vi "Get all positions.vi"(7 "JSON":string, 9 "Offset":i32) -> (1 "Offset past All":i32, 2 "Array":T2(array[cluster]), 3 "State":T3)   [LabVIEW 2017, in "JSONtext.lvlib"]
uses:
  JSONtext.lvlib
  Parsing State.ctl
  JSON Value Type.ctl
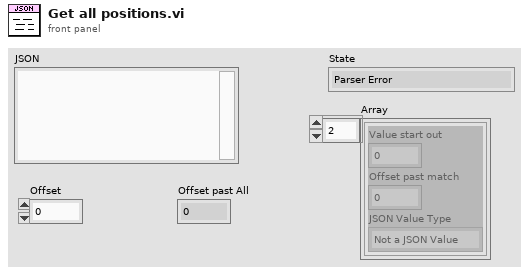
[diagram p1: front panel]
types:
  T1 = typedef "JSONtext.lvlib/JSON Value Type.ctl" = enum16{"Not a JSON Value", "JSON Object", "JSON Array", "String", "Number", "true", "false", "null"}
  T2 = cluster{"Value start out":i32, "Offset past match":i32, "JSON Value Type":T1}[]
  T3 = typedef "JSONtext.lvlib/Parsing State.ctl" = enum16{"Parser Error", "Object", "Array", "String", "Number/Other", "Leading Whitespace", "Object end", "Array end", "Value end"}
  T4 = cluster{"Value start out":i32, "Offset past match":i32, "JSON Value Type":T1}
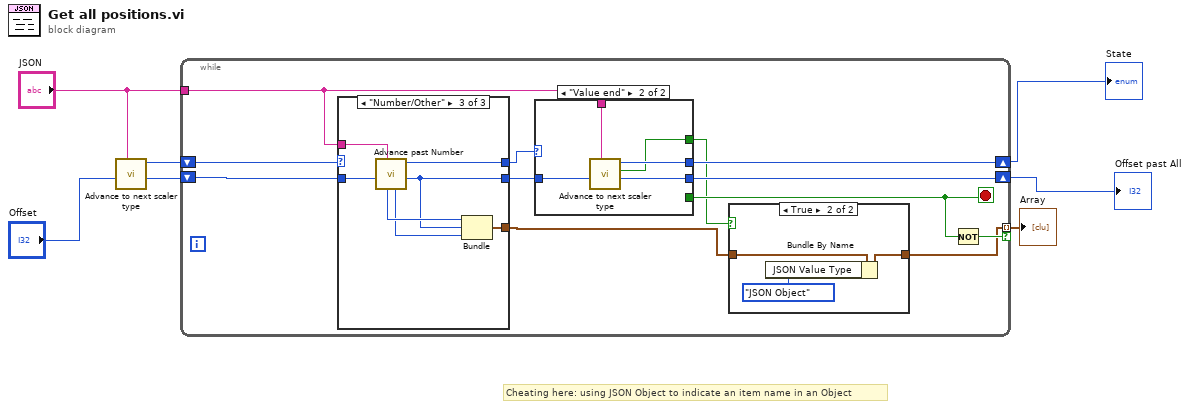
[diagram p0: block diagram]
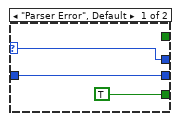
[diagram p3: hidden frame]
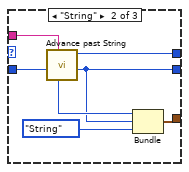
[diagram p5: hidden frame]
diagram:
  # "Cheating here: using JSON Object to indicate an item name in an Object"
  n1 = call "Advance to next scaler type.vi"("JSON"="JSON", "Offset"="Offset") -> ("Offset of first character of scaler"=w3:i32, "Parser State"=w1:T3)  [unwired: 7 in, 1 out]
  n2 = while {
    tunnel: "JSON" -> [w13]
    shift-right: [w16] -> w7
    shift-left: w3 -> [w12]
    tunnel: [w8] -> w5 mode=indexing if=w14
    shift-right: [w15] -> w6
    shift-left: w1 -> [w11]
    stop <- w17 stop-if-true
    n3 = case shown="\"Number/Other\"" w11 {
      selector: w11 -> [w33 _ _]
      tunnel: w12 -> [w32 w39 w46]
      tunnel: [w33 w40 w47] -> w18
      tunnel: [w32 w35 w43] -> w19
      tunnel: w13 -> [_ w38 w45]
      tunnel: [_ w37 w42] -> w9
      frame Default {
      }
      frame "String" {
        n4 = call "Advance past String.vi"("JSON"=w38, "Offset"=w39) -> ("Offset past match"=w35:i32, "State"=w40:T3, "Value start out"=w36:i32)  [unwired: 7 in]
        n5 = Bundle("Value start out"=w36, "Offset past match"=w35, "JSON Value Type"=JSON_Value_Type."String") -> (w37:T4)  [unwired: 1 in]
      }
      frame "Number/Other" {
        n6 = call "Advance past Number.vi"("JSON"=w45, "Offset (0)"=w46) -> ("Offset past match"=w43:i32, "Parser State"=w47:T3, "JSON Value Type"=w41:T1, "Value start out"=w44:i32)  [unwired: 6 in]
        n7 = Bundle("Value start out"=w44, "Offset past match"=w43, "JSON Value Type"=w41) -> (w42:T4)  [unwired: 1 in]
      }
    }
    n8 = case shown="\"Value end\"" w18 {
      selector: w18 -> [w24 _]
      tunnel: w19 -> [w25 w31]
      tunnel: [TRUE _] -> w17
      tunnel: [w24 w29] -> w15
      tunnel: [w25 w28] -> w16
      tunnel: w13 -> [_ w30]
      tunnel: [_ w27] -> w10
      frame "Parser Error", Default {
      }
      frame "Value end" {
        n9 = call "Advance to next scaler type.vi"("JSON"=w30, "Offset"=w31) -> ("Offset of first character of scaler"=w28:i32, "Found colon"=w27:bool, "Parser State"=w29:T3)  [unwired: 7 in]
      }
    }
    n10 = case shown="True" w10 {
      tunnel: w9 -> [w20 w23]
      tunnel: [w20 w22] -> w8
      frame False {
      }
      frame True {
        n11 = Bundle By Name(cluster=w23, "JSON Value Type"=JSON_Value_Type."JSON Object") -> (w22:T4)
      }
    }
    n12 = Not(x=w17) -> (.not. x?=w14:bool)
  }
  "State" <- w6
  "Offset past All" <- w7
  "Array" <- w5
